vi "Stop Core.vi"(10 "final error code":i32, 11 "Main in":refnum<class "Main.lvclass">) -> (3 "Main out":refnum<class "Main.lvclass">)   [LabVIEW 2015, in "Main.lvlib" / "Main.lvclass"]
doc: "(<B>Filename</B>: Actor Framework.lvlib:Actor.lvclass:Stop Core.vi)\n\nDefines what the actor does before it stops. Use the <B>final error code</B> input to determine whether the actor shut down in response to an error.\n\nBy default, this method does nothing. A descendant class may override it to define behavior, such as shutting down any processes the actor initiated in its override of the Actor Core method."
uses:
  Main.lvclass
  Main.lvclass/Main.ctl
  <vilib>/ActorFramework/Actor/Actor.lvclass
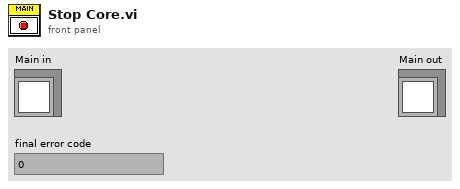
[diagram p1: front panel]
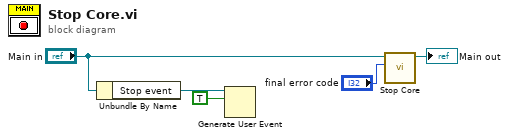
[diagram p0: block diagram]
diagram:
  n1 = Unbundle By Name("Main in") -> ("Stop event"=w2:refnum<user-event>)
  n2 = Generate User Event(user event=w2, event data cluster=TRUE ("event data")) -> ()  [unwired: 2 in, 2 out]
  n3 = call-parent "Stop Core.vi"("final error code"="final error code", "Actor in"="Main in") -> ("Actor out"=→"Main out":refnum<class "Main.lvclass">)  [unwired: 9 in]
